vi "Live_ConvertSetting_Examples.vi"() -> ()   [LabVIEW 2019]
doc: "This example demonstrates the image acquisition with one camera in ring buffer mode together with a live display of the latest images during record. After record is stopped, the images can be addressed by index.\nAdditionally the image convert settings can be adjusted at any time\nNote that this example will not be fail save, i.e. doesnt react on errors, just handles them forward to the end\n\nUsage:\nSelect your required image count and the camera setup before you start the program.\nOnce started, the camera class will be initialized and images will be recorded and displayed automatically\nYou can stop the images by pressing stop record.\nAfter stopped, the image at the selected index will be read out\nTo finish the program click on quit application, this will force an exit of the camera class\nYou can change your required ROI after and also during the record."
uses:
  camera/Camera.lvclass
  pco.sdk/TimingControl/TimingControl.lvlib
  <vilib>/picture/picture.llb/Draw True-Color Pixmap.vi
  <vilib>/picture/picture.llb/Draw 8-Bit Pixmap.vi
panel:
  out "colormap(U8)":u32[](array[numeric])
  out "Image(U16)":u16[][](graph)
  in  "Zoom [%]":i32(slide)=26 min=10 max=200 step=5 scale=10.0..200.0
  out "Image":picture
  in  "settingsChanged":bool
  in  "Trigger":bool
  in  "LUT File":path
  in  "data_format":T1(ring)=enum."RGBA8"
  in  "Auto Range":bool
  out "rawImage":u16[][](array[numeric])
  in  "iContrast [%]":i32 min=-100 max=99 step=1
  in  "Gamma":dbl=1.0 min=0.01 max=10.0 step=0.01 format="%.2f"
  in  "whiteBalance":bool
  in  "iScale_max":u16=60000 step=1
  in  "iScale_min":u16=200 step=1
  in  "Image Index":u32 max=9
  out "Recorded Images":u32
  in  "TriggerMode":T2(ring)
  in  "Quit":bool
  out "Error":errorcluster {"code" format="%x"}
  in  "Stop Record":bool
  out "Recording On":bool
  in  "cropY1":u64=2 min=1 max=2048 step=1
  in  "cropX1":u64=2 min=1 max=2048 step=1
  in  "cropY0":u64=1 min=1 max=2047 step=1
  in  "cropX0":u64=1 min=1 max=2047 step=1
  out "Image Height":u64
  out "Image Width":u64
  in  "dwImgCount":u32=10 caption="Required Number of Images" max=2397
  in  "Exposure Time [s]":dbl=0.010000000000000002 step=0.001
  # "This example demonstrates the image acquisition with one camera in ring buffer mode together with a live display of the latest images during record. After record is stopped, the images can be addressed by index.\nAdditionally the image convert settings can be adjusted at any time\nNote that this example will not be fail save, i.e. doesnt react on errors, just handles them forward to the end\n\nUsage:\nSelect your required image count and the camera setup before you start the program.\nOnce started, the camera class will be initialized and images will be recorded and displayed automatically\nYou can stop the images by pressing stop record.\nAfter stopped, the image at the selected index will be read out\nTo finish the program click on quit application, this will force an exit of the camera class\nYou can change your required ROI after and also during the record."
  # "pco.labview"
  # "Camera Setup"
  # "Recording Control"
  # "Parameters for image readout"
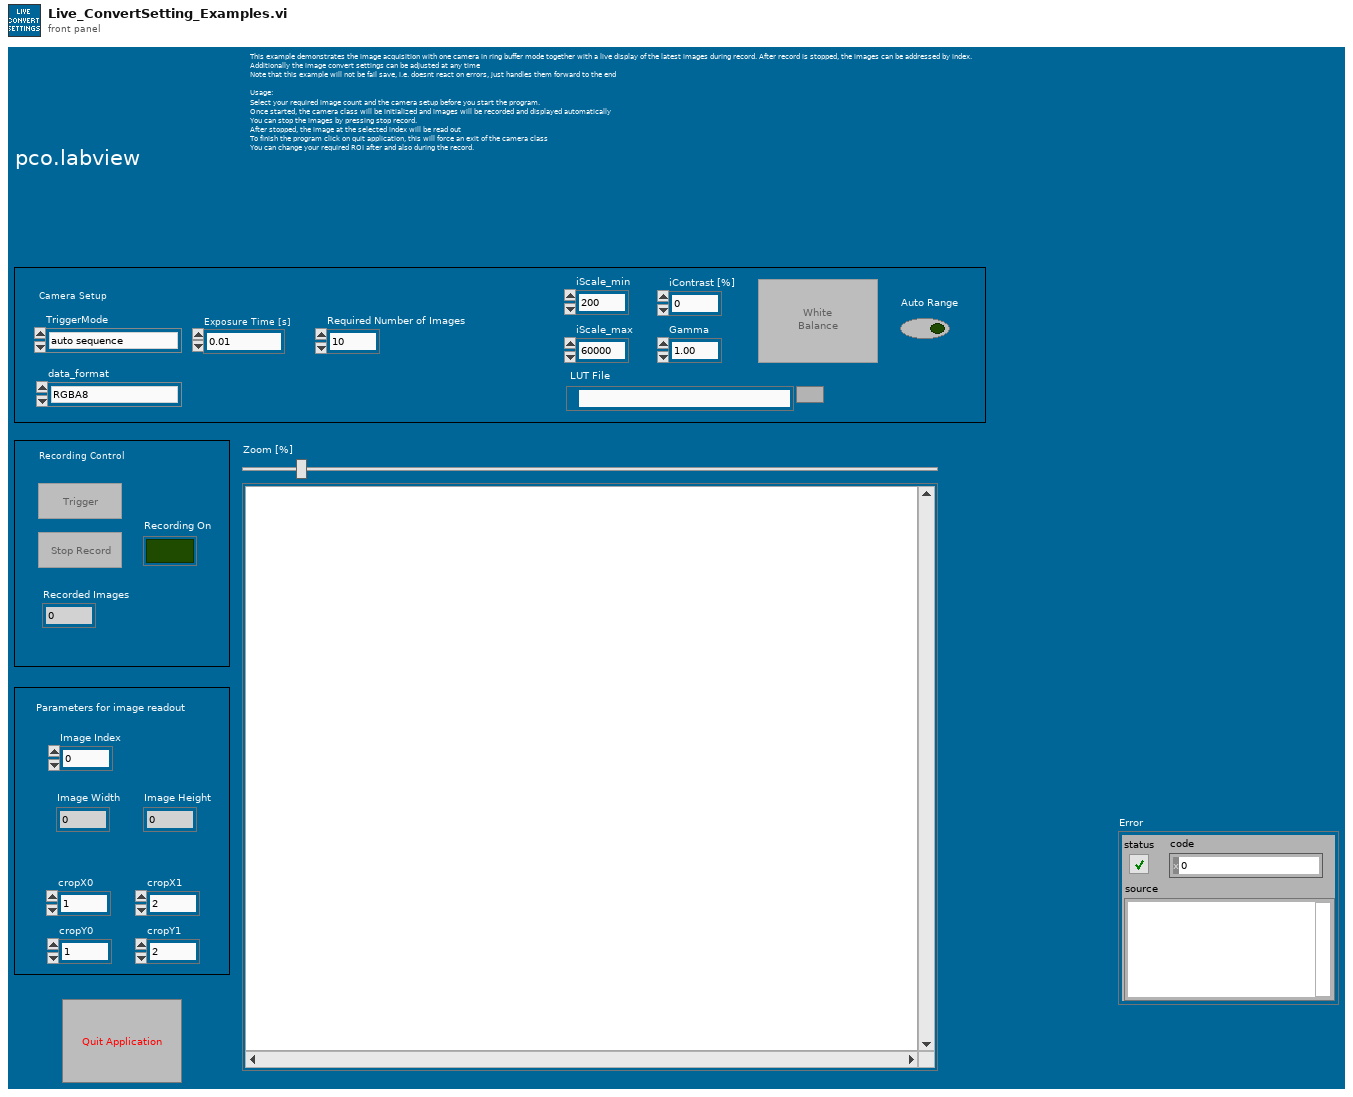
[diagram p1: front panel]
types:
  T1 = enum16{"Undefined", "Mono8", "Mono16", "BGRA8", "RGBA8", "BGRA16", "RGBA16", "CompressedMono8"}
  T2 = enum16{"auto sequence", "software trigger", "external exposure start", "external exposure control"}
  T3 = enum16{"sequence", "sequence non blocking", "ring buffer", "fifo", "tif", "multitif", "pcoraw", "b16", "dicom", "multidicom", "camram_ring", "camram_segment"}
  T4 = enum8{"Enabled", "Disabled", "Disabled and Grayed Out"}
  T5 = cluster{"serial":u32, "type":u16, "sub_type":u16, "interface_type":u16, "bit_resolution":u16, "min_exposure_time_s":dbl, "max_exposure_time_s":dbl, "min_exposure_step_s":dbl, "min_delay_time_s":dbl, "max_delay_time_s":dbl, "min_delay_step_s":dbl, "min_width":u64, "min_height":u64, "max_width":u64, "max_height":u64, "roi_step_horz":u64, "roi_step_vert":u64, "roi_symmetric_horz":bool, "roi_symmetric_vert":bool, "has_timestamp_mode":bool, "has_timestamp_mode_ascii_only":bool, "pixelrate_vec":u32[], "conversion_factor_vec":sgl[], "has_trigger_mode_extexpctrl":bool, "has_acquire_mode":bool, "has_ext_acquire_mode":bool, "has_metadata_mode":bool, "has_ram":bool, "binning_horz_vec":u16[], "binning_vert_vec":u16[], "has_average_binning":bool, "pixel_format_vec":u32[]}
  T6 = cluster{"wSignalNum":u16, "wEnabled":u16, "wType":u16, "wPolarity":u16, "wFilterSetting":u16, "wSelected":u16, "dwParameter":u32[], "dwSignalFunctionality":u32[]}
  T7 = typedef "Camera.lvclass/binning.ctl" = cluster{"vert":u16, "horz":u16, "mode":u16}
  T8 = cluster{"exposure_time_s":dbl, "delay_time_s":dbl, "roi":cluster{"x0":u64, "y0":u64, "x1":u64, "y1":u64}, "timestamp_mode":u16, "pixelrate":u32, "conversion_factor":sgl, "trigger_mode":u16, "acquire_mode":u16, "acquire_sequence_number":u32, "metadata_mode":u16, "noisefilter_mode":u16, "pixel_format":u32, "binning":T7, "auto_exposure":cluster{"region":u16, "min_exposure_s":dbl, "max_exposure_s":dbl}}
  T9 = cluster{"sharpen":bool, "adaptive_sharpen":bool, "flip_vertical":bool, "auto_minmax":bool, "add_conv_flags":u32, "min_limit":u16, "max_limit":u16, "gamma":dbl, "contrast":i32, "pco_debayer_algorithm":bool, "color_temperature":i32, "color_saturation":i32, "color_vibrance":i32, "color_tint":i32, "lut_file":path}
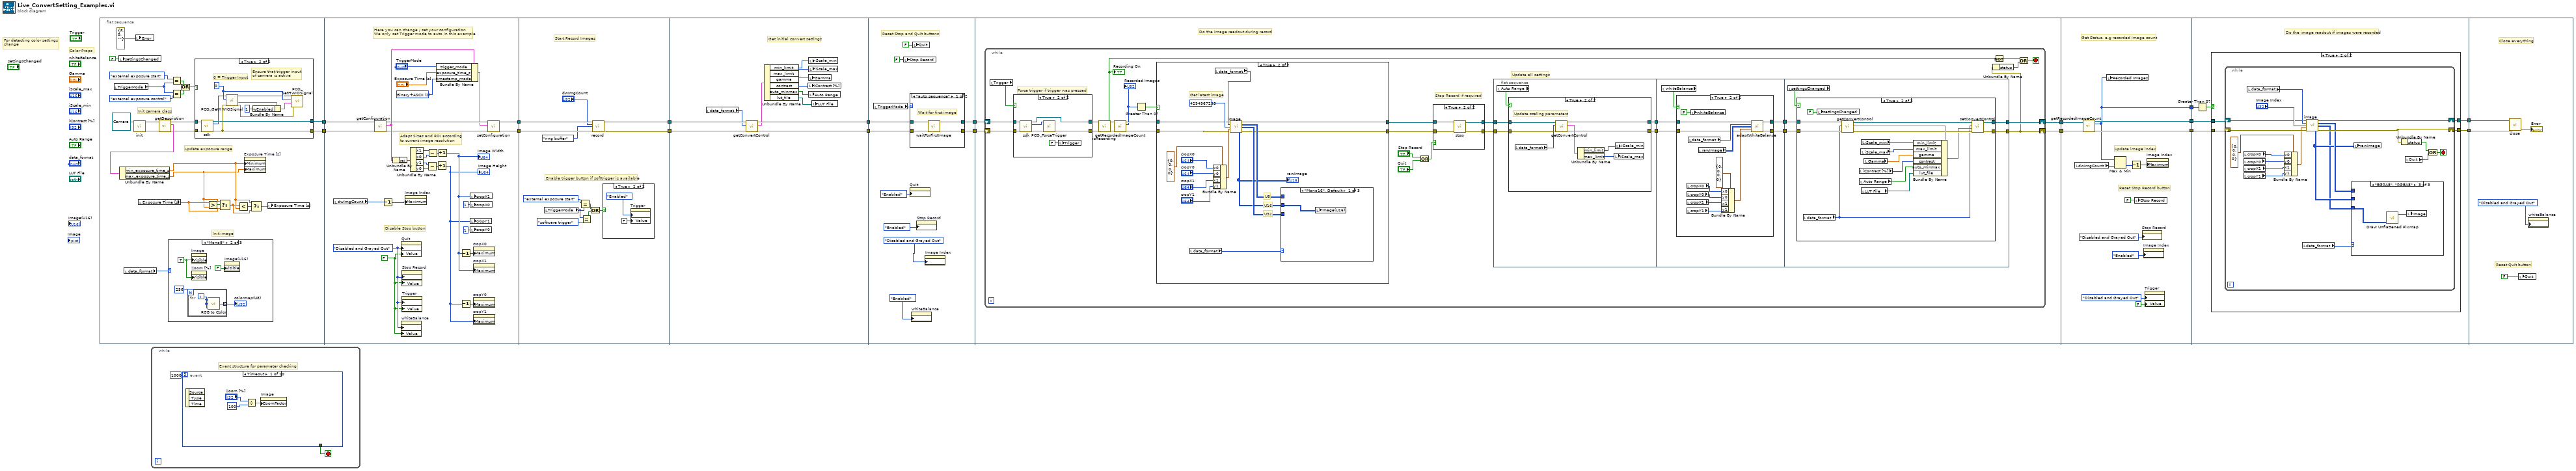
[diagram p0: block diagram]
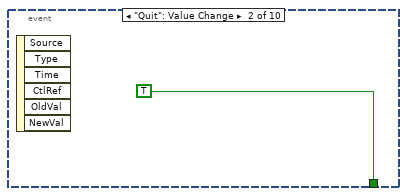
[diagram p2: hidden frame]
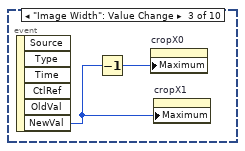
[diagram p3: hidden frame]
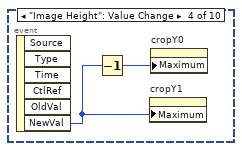
[diagram p4: hidden frame]
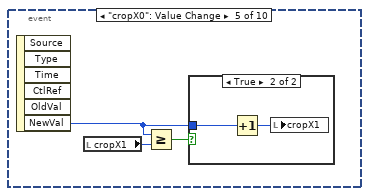
[diagram p5: hidden frame]
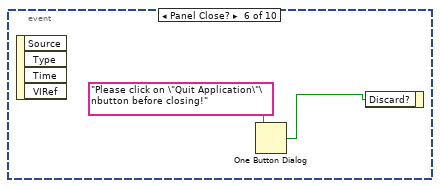
[diagram p7: hidden frame]
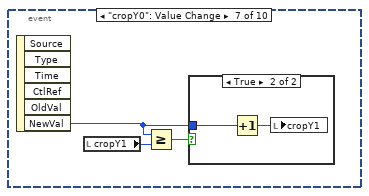
[diagram p8: hidden frame]
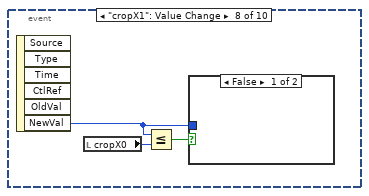
[diagram p10: hidden frame]
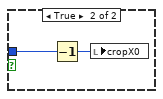
[diagram p11: hidden frame]
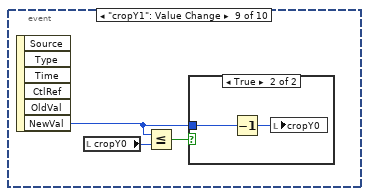
[diagram p12: hidden frame]
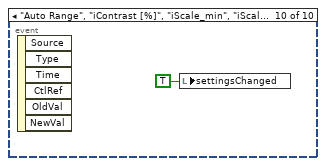
[diagram p14: hidden frame]
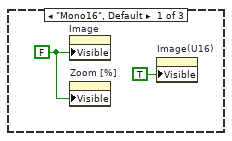
[diagram p16: hidden frame]
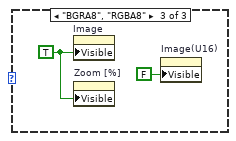
[diagram p17: hidden frame]
diagram:
  # "For detecting color settings\nchange"
  # "Color Props"
  n1 = flat-sequence {
    tunnel: [w24] -> w7
    tunnel: [w25] -> w1
    tunnel: [w69] -> w17
    tunnel: [w73] -> w16
    tunnel: w7 -> [w68]
    tunnel: w1 -> [w67]
    tunnel: w17 -> [w103]
    tunnel: w16 -> [w104]
    tunnel: [w100] -> w11
    tunnel: [w101] -> w8
    tunnel: w11 -> [w117]
    tunnel: [w112] -> w10
    tunnel: [w118] -> w9
    tunnel: w8 -> [w108]
    tunnel: w10 -> [w125]
    tunnel: w9 -> [w126]
    tunnel: [w124] -> w15
    tunnel: [w121] -> w3
    tunnel: w15 -> [w139]
    tunnel: [w138] -> w14
    tunnel: [w137] -> w6
    tunnel: w3 -> [w136]
    tunnel: w14 -> [w274]
    tunnel: [w272] -> w13
    tunnel: w6 -> [w267]
    tunnel: [w266] -> w5
    tunnel: [w265] -> w2
    tunnel: w13 -> [w283]
    tunnel: [w282] -> w12
    tunnel: w5 -> [w281]
    tunnel: [w280] -> w4
    tunnel: w2 -> [w278]
    tunnel: w12 -> [w318]
    tunnel: w4 -> [w315]
    frame #0 {
      # "Init image"
      # "Init camera class"
      # "Update exposure range"
      n2 = local read "TriggerMode"() -> (w18:T2)
      n3 = local write "settingsChanged"(FALSE ("settingsChanged")) -> ()
      n4 = local read "data_format"() -> (w29:T1)
      n5 = call-dynamic "init.vi"("Camera in"=refnum<class "Camera.lvclass"> refnum) -> ("Camera out"=w33:refnum<class "Camera.lvclass">, "error out"=w34:errorcluster)  [unwired: 8 in]
      n6 = local write "Error"(errorcluster {"status"=FALSE, "code"=0, "source"=""} ("error IO")) -> ()
      n7 = local read "Exposure Time [s]"() -> (w40:dbl)
      n8 = call-dynamic "getDescription.vi"("error in (no error)"=w34, "Camera in"=w33) -> ("error out"=w26:errorcluster, "description"=w32:T5, "Camera out"=w27:refnum<class "Camera.lvclass">)  [unwired: 7 in]
      n9 = Unbundle By Name(w32) -> ("min_exposure_time_s"=w31:dbl, "max_exposure_time_s"=w30:dbl)
      n10 = case shown="\"Mono8\"" w29 {
        frame "Mono16", Default {
          w55 = FALSE ("Visible")
          n11 = property on="Image" class="Pict"("Visible"=w55) -> ()  [unwired: 2 in, 2 out]
          n12 = property on="Zoom [%]" class="Slide (strict)"("Visible"=w55) -> ()  [unwired: 2 in, 2 out]
          n13 = property on="Image(U16)" class="IntGraph (strict)"("Visible"=TRUE) -> ()  [unwired: 2 in, 2 out]
        }
        frame "Mono8" {
          w57 = TRUE ("Visible")
          n14 = for {
            N: 256 -> [_]
            tunnel: [w61] -> w60 mode=indexing
            i -> [w62]
            n15 = call <vilib>:"RGB to Color.vi"("B"=w62, "G"=w62, "R"=w62) -> ("Color"=w61:u32)
          }
          "colormap(U8)" <- w60
          n16 = property on="Image" class="Pict"("Visible"=w57) -> ()  [unwired: 2 in, 2 out]
          n17 = property on="Zoom [%]" class="Slide (strict)"("Visible"=w57) -> ()  [unwired: 2 in, 2 out]
          n18 = property on="Image(U16)" class="IntGraph (strict)"("Visible"=FALSE) -> ()  [unwired: 2 in, 2 out]
        }
        frame "BGRA8", "RGBA8" {
          w63 = TRUE ("Visible")
          n19 = property on="Image" class="Pict"("Visible"=w63) -> ()  [unwired: 2 in, 2 out]
          n20 = property on="Zoom [%]" class="Slide (strict)"("Visible"=w63) -> ()  [unwired: 2 in, 2 out]
          n21 = property on="Image(U16)" class="IntGraph (strict)"("Visible"=FALSE) -> ()  [unwired: 2 in, 2 out]
        }
      }
      n22 = Equal?(x=T2."external exposure start" ("TriggerMode"), y=w18) -> (x = y?=w22:bool)
      n23 = Equal?(x=w18, y=T2."external exposure control" ("TriggerMode")) -> (x = y?=w21:bool)
      n24 = Or(x=w22, y=w21) -> (x .or. y?=w20:bool)
      n25 = case shown="True" w20 {
        tunnel: w27 -> [w43 w47]
        tunnel: w26 -> [w42 w46]
        tunnel: [w42 w44] -> w25
        tunnel: [w43 w45] -> w24
        frame False {
        }
        frame True {
          w52 = u16 0 ("wSignalNum")
          # "0 = Trigger Input"
          # "Ensure that trigger input\nof camera is active"
          n26 = call-dynamic "sdk.vi"("Camera in"=w47, "error in (no error)"=w46) -> ("Camera out"=w45:refnum<class "Camera.lvclass">, "sdk"=w48:u64, "error out"=w44:errorcluster)  [unwired: 11 in]
          n27 = call "PCO_GetHWIOSignal.vi"("error in (no error)"=w44, "wSignalNum"=w52, "ph"=w48) -> ("error out"=w50:errorcluster, "strSignal"=w54:T6, "ph out"=w49:u64)  [unwired: 5 in, 1 out]
          n28 = Bundle By Name(cluster=w54, "wEnabled"=u16 1) -> (w51:T6)
          n29 = call "PCO_SetHWIOSignal.vi"("error in (no error)"=w50, "strSignal"=w51, "wSignalNum"=w52, "ph"=w49) -> ()  [unwired: 5 in, 3 out]
        }
      }
      n30 = Greater?(x=w40, y=w30) -> (0:w41:bool)
      n31 = Select(t=w30, s=w41, f=w40) -> (s? t:f=w38:dbl)
      n32 = Less?(x=w38, y=w31) -> (x < y?=w39:bool)
      n33 = property on="Exposure Time [s]" class="DigNum (strict)"("Minimum"=w31, "Maximum"=w30) -> ()  [unwired: 2 in, 2 out]
      n34 = Select(t=w31, s=w39, f=w38) -> (s? t:f=w37:dbl)
      n35 = local write "Exposure Time [s]"(w37) -> ()
    }
    frame #1 {
      w79 = u16 2 items=["OFF", "Binary", "Binary+ASCII", "ASCII"] ("wTimeStampMode")
      w65 = FALSE ("Stop")
      w66 = T4."Disabled and Grayed Out" ("Disabled")
      # "Disable Stop button"
      # "Adapt Sizes and ROI according\nto current image resolution"
      # "Here you can change / set your configuration\nWe only set Trigger mode to auto in this example"
      n36 = local read "dwImgCount"() -> (w80:u32)
      n37 = call-dynamic "getConfiguration.vi"("error in (no error)"=w67, "Camera in"=w68) -> ("error out"=w74:errorcluster, "configuration"=w85:T8, "Camera out"=w76:refnum<class "Camera.lvclass">)  [unwired: 7 in]
      n38 = Decrement(x=w80) -> (x-1=w70:u32)
      n39 = Unbundle By Name(w85) -> ("roi"=w86:cluster{"x0":u64, "y0":u64, "x1":u64, "y1":u64})
      n40 = property on="Quit" class="Bool (strict)"("DisabledEnum"=w66, "Value"=w65) -> ()  [unwired: 2 in, 2 out]
      n41 = property on="whiteBalance" class="Bool (strict)"("DisabledEnum"=w66, "Value"=w65) -> ()  [unwired: 2 in, 2 out]
      n42 = property on="Stop Record" class="Bool (strict)"("DisabledEnum"=w66, "Value"=w65) -> ()  [unwired: 2 in, 2 out]
      n43 = property on="Trigger" class="Bool (strict)"("DisabledEnum"=w66, "Value"=w65) -> ()  [unwired: 2 in, 2 out]
      n44 = property on="Image Index" class="DigNum (strict)"("Maximum"=w70) -> ()  [unwired: 2 in, 2 out]
      n45 = Unbundle By Name(w86) -> ("x1"=w88:u64, "x0"=w87:u64, "y1"=w90:u64, "y0"=w89:u64)
      n46 = Subtract(x=w90, y=w89) -> (x-y=w92:u64)
      n47 = Subtract(x=w88, y=w87) -> (x-y=w91:u64)
      n48 = Bundle By Name(cluster=w85, "trigger_mode"="TriggerMode", "exposure_time_s"="Exposure Time [s]", "timestamp_mode"=w79) -> (w75:T8)
      n49 = Increment(x=w92) -> (x+1=w71:u64)
      "Image Height" <- w71
      n50 = Increment(x=w91) -> (x+1=w72:u64)
      "Image Width" <- w72
      n51 = Decrement(x=w72) -> (x-1=w83:u64)
      n52 = Decrement(x=w71) -> (x-1=w84:u64)
      n53 = local write "cropX1"(w72) -> ()
      n54 = local write "cropX0"(u64 1 ("roiY0")) -> ()
      n55 = local write "cropY1"(w71) -> ()
      n56 = local write "cropY0"(u64 1 ("roiY0")) -> ()
      n57 = property on="cropX0" class="DigNum (strict)"("Maximum"=w83) -> ()  [unwired: 2 in, 2 out]
      n58 = property on="cropX1" class="DigNum (strict)"("Maximum"=w72) -> ()  [unwired: 2 in, 2 out]
      n59 = property on="cropY0" class="DigNum (strict)"("Maximum"=w84) -> ()  [unwired: 2 in, 2 out]
      n60 = property on="cropY1" class="DigNum (strict)"("Maximum"=w71) -> ()  [unwired: 2 in, 2 out]
      n61 = call-dynamic "setConfiguration.vi"("error in (no error)"=w74, "configuration"=w75, "Camera in"=w76) -> ("error out"=w73:errorcluster, "Camera out"=w69:refnum<class "Camera.lvclass">)  [unwired: 7 in]
    }
    frame #2 {
      # "Enable trigger button if softtrigger is available"
      # "Start Record Images"
      n62 = local read "TriggerMode"() -> (w98:T2)
      n63 = Equal?(x=T2."external exposure start" ("TriggerMode"), y=w98) -> (x = y?=w95:bool)
      n64 = Equal?(x=w98, y=T2."software trigger" ("TriggerMode")) -> (x = y?=w94:bool)
      n65 = Or(x=w95, y=w94) -> (x .or. y?=w96:bool)
      n66 = call-dynamic "record.vi"("Camera in"=w103, "num_images"="dwImgCount", "record_mode"=T3."ring buffer", "error in (no error)"=w104) -> ("Camera out"=w101:refnum<class "Camera.lvclass">, "error out"=w100:errorcluster)  [unwired: 10 in]
      n67 = case shown="True" w96 {
        frame False {
        }
        frame True {
          n68 = property on="Trigger" class="Bool (strict)"("DisabledEnum"=T4."Enabled" ("Disabled"), "Value"=FALSE ("Trigger")) -> ()  [unwired: 2 in, 2 out]
        }
      }
    }
    frame #3 {
      # "Get initial convert settings"
      n69 = local read "data_format"() -> (w107:T1)
      n70 = call-dynamic "getConvertControl.vi"("error in (no error)"=w117, "data_format"=w107, "Camera in"=w108) -> ("error out"=w112:errorcluster, "convert_control"=w116:T9, "Camera out"=w118:refnum<class "Camera.lvclass">)  [unwired: 6 in]
      n71 = Unbundle By Name(w116) -> ("min_limit"=w114:u16, "max_limit"=w113:u16, "gamma"=w115:dbl, "contrast"=w111:i32, "auto_minmax"=w110:bool, "lut_file"=w109:path)
      n72 = local write "iContrast [%]"(w111) -> ()
      n73 = local write "Gamma"(w115) -> ()
      n74 = local write "iScale_min"(w114) -> ()
      n75 = local write "iScale_max"(w113) -> ()
      n76 = local write "Auto Range"(w110) -> ()
      n77 = local write "LUT File"(w109) -> ()
    }
    frame #4 {
      # "Reset Stop and Quit buttons"
      n78 = local read "TriggerMode"() -> (w119:T2)
      n79 = local write "Stop Record"(FALSE ("Stop Record")) -> ()
      n80 = case shown="\"auto sequence\"" w119 {
        tunnel: w126 -> [w133 w135]
        tunnel: w125 -> [w132 w134]
        tunnel: [w131 w134] -> w124
        tunnel: [w130 w135] -> w121
        frame "auto sequence" {
          # "Wait for first image"
          n81 = call-dynamic "waitForFirstImage.vi"("error in (no error)"=w132, "Camera in"=w133) -> ("error out"=w131:errorcluster, "Camera out"=w130:refnum<class "Camera.lvclass">)  [unwired: 8 in]
        }
        frame Default {
          # "Don't wait \nif we trigger"
        }
      }
      n82 = property on="Quit" class="Bool (strict)"("DisabledEnum"=T4."Enabled" ("Disabled")) -> ()  [unwired: 2 in, 2 out]
      n83 = property on="whiteBalance" class="Bool (strict)"("DisabledEnum"=T4."Enabled" ("Disabled")) -> ()  [unwired: 2 in, 2 out]
      n84 = local write "Quit"(FALSE ("Stop")) -> ()
      n85 = property on="Stop Record" class="Bool (strict)"("DisabledEnum"=T4."Enabled" ("Disabled")) -> ()  [unwired: 2 in, 2 out]
      n86 = property on="Image Index" class="DigNum (strict)"("DisabledEnum"=T4."Disabled and Grayed Out" ("Disabled")) -> ()  [unwired: 2 in, 2 out]
    }
    frame #5 {
      # "Do the image readout during record"
      n87 = while {
        shift-right: [w149] -> w138
        shift-left: w139 -> [w152]
        shift-right: [w155] -> w137
        shift-left: w136 -> [w153]
        stop <- w167 stop-if-true
        # "Stop Record if required"
        # "Force trigger if trigger was pressed"
        # "Update all settings"
        n88 = local read "Trigger"() -> (w154:bool)
        n89 = case shown="True" w154 {
          tunnel: w153 -> [w199 w204]
          tunnel: w152 -> [w198 w203]
          tunnel: [w199 w202] -> w151
          tunnel: [w198 w201] -> w150
          frame False {
          }
          frame True {
            n90 = call-dynamic "sdk.vi"("Camera in"=w204, "error in (no error)"=w203) -> ("Camera out"=w202:refnum<class "Camera.lvclass">, "sdk"=w205:u64, "error out"=w206:errorcluster)  [unwired: 11 in]
            n91 = call "PCO_ForceTrigger.vi"("error in (no error)"=w206, "ph"=w205) -> ("error out"=w201:errorcluster)  [unwired: 6 in, 3 out]
            n92 = local write "Trigger"(FALSE ("Trigger")) -> ()
          }
        }
        n93 = call-dynamic "isRecording.vi"("Camera in"=w151, "error in (no error)"=w150) -> ("Camera out"=w163:refnum<class "Camera.lvclass">, "recording"=w165:bool, "error out"=w162:errorcluster)  [unwired: 11 in]
        "Recording On" <- w165
        n94 = call-dynamic "getRecordedImageCount.vi"("Camera in"=w163, "error in (no error)"=w162) -> ("Camera out"=w160:refnum<class "Camera.lvclass">, "recorded_image_count"=w148:u32, "error out"=w161:errorcluster)  [unwired: 11 in]
        "Recorded Images" <- w148
        n95 = Greater Than 0?(x=w148) -> (x > 0?=w147:bool)
        n96 = case shown="True" w147 {
          tunnel: w161 -> [w174 w184]
          tunnel: w160 -> [w175 w178]
          tunnel: [w174 w176] -> w143
          tunnel: [w175 w177] -> w142
          frame False {
          }
          frame True {
            # "U32"
            # "U8"
            # "U16"
            # "Get latest image"
            n97 = local read "data_format"() -> (w179:T1)
            n98 = Bundle By Name(cluster=cluster{"x0":u64, "y0":u64, "x1":u64, "y1":u64} {"x0"=0, "y0"=0, "x1"=0, "y1"=0} ("roi"), "x0"="cropX0", "y0"="cropY0", "x1"="cropX1", "y1"="cropY1") -> (w187:cluster{"x0":u64, "y0":u64, "x1":u64, "y1":u64})
            n99 = local read "data_format"() -> (w183:T1)
            n100 = call-dynamic "image.vi"("Camera in"=w178, "data_format"=w183, "image_index"=u32 4294967295 ("dwImgIdx"), "crop"=w187, "error in (no error)"=w184) -> ("Camera out"=w177:refnum<class "Camera.lvclass">, "image (U8)"=w181:u8[][], "image (U32)"=w182:u32[][], "raw_image (U16)"=w180:u16[][], "error out"=w176:errorcluster)  [unwired: 2 in, 4 out]
            "rawImage" <- w180
            n101 = case shown="\"Mono16\", Default" w179 {
              tunnel: w182 -> [_ _ w197]
              tunnel: w181 -> [_ w194 _]
              tunnel: w180 -> [w192 _ _]
              frame "Mono16", Default {
                n102 = local write "Image(U16)"(w192) -> ()
              }
              frame "Mono8" {
                n103 = local read "colormap(U8)"() -> (w193:u32[])
                n104 = call-poly <vilib>:"Draw Unflattened Pixmap.vi"("data"=w194, "color table"=w193) -> ("new picture"=w195:picture)  [unwired: 7 in]
                n105 = local write "Image"(w195) -> ()
              }
              frame "BGRA8", "RGBA8" {
                n106 = call-poly <vilib>:"Draw Unflattened Pixmap.vi"("data (RGB format)"=w197) -> ("new picture"=w196:picture)  [unwired: 8 in]
                n107 = local write "Image"(w196) -> ()
              }
            }
          }
        }
        n108 = Or(x="Stop Record", y="Quit") -> (x .or. y?=w146:bool)
        n109 = case shown="True" w146 {
          tunnel: w143 -> [w169 w170]
          tunnel: [w168 w172] -> w141
          tunnel: [w169 w173] -> w140
          tunnel: w142 -> [w168 w171]
          frame False {
          }
          frame True {
            n110 = call-dynamic "stop.vi"("error in (no error)"=w170, "Camera in"=w171) -> ("error out"=w173:errorcluster, "Camera out"=w172:refnum<class "Camera.lvclass">)  [unwired: 8 in]
          }
        }
        n111 = flat-sequence {
          tunnel: w140 -> [w209]
          tunnel: w141 -> [w210]
          tunnel: [w208] -> w159
          tunnel: [w207] -> w158
          tunnel: w159 -> [w225]
          tunnel: w158 -> [w224]
          tunnel: [w223] -> w157
          tunnel: [w222] -> w156
          tunnel: w157 -> [w244]
          tunnel: w156 -> [w245]
          tunnel: [w243] -> w149
          tunnel: [w242] -> w155
          frame #0 {
            n112 = local read "Auto Range"() -> (w211:bool)
            n113 = case shown="True" w211 {
              tunnel: w210 -> [w213 w217]
              tunnel: w209 -> [w212 w216]
              tunnel: [w212 w215] -> w208
              tunnel: [w213 w214] -> w207
              frame False {
              }
              frame True {
                # "Update scaling parameters"
                n114 = local read "data_format"() -> (w221:T1)
                n115 = call-dynamic "getConvertControl.vi"("error in (no error)"=w216, "data_format"=w221, "Camera in"=w217) -> ("error out"=w215:errorcluster, "convert_control"=w218:T9, "Camera out"=w214:refnum<class "Camera.lvclass">)  [unwired: 6 in]
                n116 = Unbundle By Name(w218) -> ("min_limit"=w219:u16, "max_limit"=w220:u16)
                n117 = local write "iScale_max"(w220) -> ()
                n118 = local write "iScale_min"(w219) -> ()
              }
            }
          }
          frame #1 {
            n119 = local read "whiteBalance"() -> (w226:bool)
            n120 = case shown="True" w226 {
              tunnel: w225 -> [w227 w233]
              tunnel: w224 -> [w228 w232]
              tunnel: [w227 w231] -> w223
              tunnel: [w228 w230] -> w222
              frame False {
              }
              frame True {
                n121 = local read "cropX0"() -> (w238:u64)
                n122 = local read "cropY0"() -> (w237:u64)
                n123 = local read "cropX1"() -> (w236:u64)
                n124 = local read "cropY1"() -> (w229:u64)
                n125 = local read "data_format"() -> (w240:T1)
                n126 = local write "whiteBalance"(FALSE ("whiteBalance")) -> ()
                n127 = local read "rawImage"() -> (w239:u16[][])
                n128 = Bundle By Name(cluster=cluster{"x0":u64, "y0":u64, "x1":u64, "y1":u64} {"x0"=0, "y0"=0, "x1"=0, "y1"=0} ("roi"), "x0"=w238, "y0"=w237, "x1"=w236, "y1"=w229) -> (w235:cluster{"x0":u64, "y0":u64, "x1":u64, "y1":u64})
                n129 = call-dynamic "adaptWhiteBalance.vi"("Camera in"=w232, "data_format"=w240, "raw_image (U16)"=w239, "roi"=w235, "error in (no error)"=w233) -> ("Camera out"=w230:refnum<class "Camera.lvclass">, "error out"=w231:errorcluster)  [unwired: 9 in]
              }
            }
          }
          frame #2 {
            n130 = local read "settingsChanged"() -> (w246:bool)
            n131 = case shown="True" w246 {
              tunnel: w245 -> [w248 w254]
              tunnel: w244 -> [w247 w253]
              tunnel: [w247 w250] -> w243
              tunnel: [w248 w249] -> w242
              frame False {
              }
              frame True {
                n132 = local read "data_format"() -> (w252:T1)
                n133 = local write "settingsChanged"(FALSE ("whiteBalance")) -> ()
                n134 = call-dynamic "getConvertControl.vi"("error in (no error)"=w253, "data_format"=w252, "Camera in"=w254) -> ("error out"=w256:errorcluster, "convert_control"=w263:T9, "Camera out"=w257:refnum<class "Camera.lvclass">)  [unwired: 6 in]
                n135 = local read "iContrast [%]"() -> (w259:i32)
                n136 = local read "Auto Range"() -> (w258:bool)
                n137 = local read "iScale_max"() -> (w261:u16)
                n138 = local read "iScale_min"() -> (w262:u16)
                n139 = local read "LUT File"() -> (w251:path)
                n140 = local read "Gamma"() -> (w260:dbl)
                n141 = Bundle By Name(cluster=w263, "min_limit"=w262, "max_limit"=w261, "gamma"=w260, "contrast"=w259, "auto_minmax"=w258, "lut_file"=w251) -> (w255:T9)
                n142 = call-dynamic "setConvertControl.vi"("error in (no error)"=w256, "convert_control"=w255, "data_format"=w252, "Camera in"=w257) -> ("error out"=w250:errorcluster, "Camera out"=w249:refnum<class "Camera.lvclass">)  [unwired: 6 in]
              }
            }
          }
        }
        n143 = Unbundle By Name(w149) -> ("status"=w166:bool)
        n144 = Not(x=w165) -> (.not. x?=w164:bool)
        n145 = Or(x=w164, y=w166) -> (x .or. y?=w167:bool)
      }
    }
    frame #6 {
      # "Update image index"
      # "Reset Stop Record button"
      # "Get Status, e.g recorded image count"
      n146 = local read "dwImgCount"() -> (w273:u32)
      n147 = call-dynamic "getRecordedImageCount.vi"("Camera in"=w267, "error in (no error)"=w274) -> ("Camera out"=w266:refnum<class "Camera.lvclass">, "recorded_image_count"=w265:u32, "error out"=w272:errorcluster)  [unwired: 11 in]
      n148 = local write "Recorded Images"(w265) -> ()
      n149 = Max & Min(x=w265, y=w273) -> (min(x,y)=w275:u32)  [unwired: 1 out]
      n150 = Decrement(x=w275) -> (x-1=w270:u32)
      n151 = local write "Stop Record"(FALSE ("Stop Record")) -> ()
      n152 = property on="Stop Record" class="Bool (strict)"("DisabledEnum"=T4."Disabled and Grayed Out" ("Disabled")) -> ()  [unwired: 2 in, 2 out]
      n153 = property on="Image Index" class="DigNum (strict)"("DisabledEnum"=T4."Enabled" ("Disabled")) -> ()  [unwired: 2 in, 2 out]
      n154 = property on="Trigger" class="Bool (strict)"("DisabledEnum"=T4."Disabled and Grayed Out" ("Disabled"), "Value"=FALSE ("Trigger")) -> ()  [unwired: 2 in, 2 out]
      n155 = property on="Image Index" class="DigNum (strict)"("Maximum"=w270) -> ()  [unwired: 2 in, 2 out]
    }
    frame #7 {
      # "Do the image readout if images were recorded"
      n156 = Greater Than 0?(x=w278) -> (x > 0?=w279:bool)
      n157 = case shown="True" w279 {
        tunnel: w283 -> [w284 w289]
        tunnel: [w284 w288] -> w282
        tunnel: w281 -> [w285 w287]
        tunnel: [w285 w286] -> w280
        frame False {
        }
        frame True {
          n158 = while {
            shift-right: [w300] -> w288
            shift-left: w289 -> [w308]
            shift-right: [w294] -> w286
            shift-left: w287 -> [w295]
            stop <- w302 stop-if-true
            n159 = local read "cropX0"() -> (w298:u64)
            n160 = local read "cropY0"() -> (w299:u64)
            n161 = local read "cropX1"() -> (w306:u64)
            n162 = local read "cropY1"() -> (w305:u64)
            n163 = local read "data_format"() -> (w296:T1)
            n164 = Bundle By Name(cluster=cluster{"x0":u64, "y0":u64, "x1":u64, "y1":u64} {"x0"=0, "y0"=0, "x1"=0, "y1"=0} ("roi"), "x0"=w298, "y0"=w299, "x1"=w306, "y1"=w305) -> (w307:cluster{"x0":u64, "y0":u64, "x1":u64, "y1":u64})
            n165 = local read "data_format"() -> (w290:T1)
            n166 = call-dynamic "image.vi"("Camera in"=w295, "data_format"=w296, "image_index"="Image Index", "crop"=w307, "error in (no error)"=w308) -> ("Camera out"=w294:refnum<class "Camera.lvclass">, "image (U8)"=w293:u8[][], "image (U32)"=w291:u32[][], "raw_image (U16)"=w292:u16[][], "error out"=w300:errorcluster)  [unwired: 2 in, 4 out]
            n167 = case shown="\"BGRA8\", \"RGBA8\"" w290 {
              tunnel: w291 -> [_ _ w314]
              tunnel: w293 -> [_ w311 _]
              tunnel: w292 -> [w309 _ _]
              frame "Mono16", Default {
                n168 = local write "Image(U16)"(w309) -> ()
              }
              frame "Mono8" {
                n169 = local read "colormap(U8)"() -> (w310:u32[])
                n170 = call-poly <vilib>:"Draw Unflattened Pixmap.vi"("data"=w311, "color table"=w310) -> ("new picture"=w312:picture)  [unwired: 7 in]
                n171 = local write "Image"(w312) -> ()
              }
              frame "BGRA8", "RGBA8" {
                n172 = call-poly <vilib>:"Draw Unflattened Pixmap.vi"("data (RGB format)"=w314) -> ("new picture"=w313:picture)  [unwired: 8 in]
                n173 = local write "Image"(w313) -> ()
              }
            }
            n174 = local write "rawImage"(w292) -> ()
            n175 = Unbundle By Name(w300) -> ("status"=w303:bool)
            n176 = local read "Quit"() -> (w304:bool)
            n177 = Or(x=w303, y=w304) -> (x .or. y?=w302:bool)
          }
        }
      }
    }
    frame #8 {
      # "Close everything"
      # "Reset Quit button"
      n178 = call-dynamic "close.vi"("error in (no error)"=w318, "Camera in"=w315) -> ("error out"=→"Error":errorcluster)  [unwired: 9 in]
      n179 = local write "Quit"(FALSE ("Stop Record")) -> ()
      n180 = property on="whiteBalance" class="Bool (strict)"("DisabledEnum"=T4."Disabled and Grayed Out" ("Disabled")) -> ()  [unwired: 2 in, 2 out]
    }
  }
  n181 = while {
    stop <- w320 stop-if-true
    # "Event structure for parameter checking"
    n182 = event shown="[0] Timeout" {
      selector: _ -> [_ _ _ _ _ _ _ _ _ _]
      dyn-events: _ -> [_ _ _ _ _ _ _ _ _ _]
      timeout: 1000 -> [_ _ _ _ _ _ _ _ _ _]
      tunnel: [_ TRUE _ _ _ _ _ _ _ _] -> w320
      event Timeout {
        n183 = event-data() -> ()  [unwired: 1 in, 3 out]
        n184 = Divide(x="Zoom [%]", y=100 ("Zoom [%]")) -> (x/y=w324:dbl)
        n185 = property on="Image" class="Pict"("ZoomFactor"=w324) -> ()  [unwired: 2 in, 2 out]
      }
      event "Quit": Value Change {
        n186 = event-data() -> ()  [unwired: 1 in, 6 out]
      }
      event "Image Width": Value Change {
        n187 = event-data() -> ("NewVal"=w326:u64)  [unwired: 1 in, 5 out]
        n188 = Decrement(x=w326) -> (x-1=w327:u64)
        n189 = property on="cropX0" class="DigNum (strict)"("Maximum"=w327) -> ()  [unwired: 2 in, 2 out]
        n190 = property on="cropX1" class="DigNum (strict)"("Maximum"=w326) -> ()  [unwired: 2 in, 2 out]
      }
      event "Image Height": Value Change {
        n191 = event-data() -> ("NewVal"=w328:u64)  [unwired: 1 in, 5 out]
        n192 = Decrement(x=w328) -> (x-1=w329:u64)
        n193 = property on="cropY1" class="DigNum (strict)"("Maximum"=w328) -> ()  [unwired: 2 in, 2 out]
        n194 = property on="cropY0" class="DigNum (strict)"("Maximum"=w329) -> ()  [unwired: 2 in, 2 out]
      }
      event "cropX0": Value Change {
        n195 = event-data() -> ("NewVal"=w330:u64)  [unwired: 1 in, 5 out]
        n196 = local read "cropX1"() -> (w332:u64)
        n197 = Greater Or Equal?(x=w330, y=w332) -> (x >= y?=w331:bool)
        n198 = case shown="True" w331 {
          tunnel: w330 -> [_ w334]
          frame False {
          }
          frame True {
            n199 = Increment(x=w334) -> (x+1=w333:u64)
            n200 = local write "cropX1"(w333) -> ()
          }
        }
      }
      event Panel Close? {
        n201 = event-data() -> ()  [unwired: 1 in, 4 out]
        n202 = One Button Dialog(message="Please click on \"Quit Application\"\nbutton before closing!") -> (true=w335:bool)  [unwired: 1 in]
        n203 = event-data("Discard?"=w335) -> ()  [unwired: 1 in, 1 out]
      }
      event "cropY0": Value Change {
        n204 = event-data() -> ("NewVal"=w337:u64)  [unwired: 1 in, 5 out]
        n205 = local read "cropY1"() -> (w339:u64)
        n206 = Greater Or Equal?(x=w337, y=w339) -> (x >= y?=w338:bool)
        n207 = case shown="True" w338 {
          tunnel: w337 -> [_ w341]
          frame False {
          }
          frame True {
            n208 = Increment(x=w341) -> (x+1=w340:u64)
            n209 = local write "cropY1"(w340) -> ()
          }
        }
      }
      event "cropX1": Value Change {
        n210 = event-data() -> ("NewVal"=w342:u64)  [unwired: 1 in, 5 out]
        n211 = local read "cropX0"() -> (w344:u64)
        n212 = Less Or Equal?(x=w342, y=w344) -> (x <= y?=w343:bool)
        n213 = case shown="False" w343 {
          tunnel: w342 -> [_ w346]
          frame False {
          }
          frame True {
            n214 = Decrement(x=w346) -> (x-1=w345:u64)
            n215 = local write "cropX0"(w345) -> ()
          }
        }
      }
      event "cropY1": Value Change {
        n216 = event-data() -> ("NewVal"=w347:u64)  [unwired: 1 in, 5 out]
        n217 = local read "cropY0"() -> (w349:u64)
        n218 = Less Or Equal?(x=w347, y=w349) -> (x <= y?=w348:bool)
        n219 = case shown="True" w348 {
          tunnel: w347 -> [_ w351]
          frame False {
          }
          frame True {
            n220 = Decrement(x=w351) -> (x-1=w350:u64)
            n221 = local write "cropY0"(w350) -> ()
          }
        }
      }
      event "Auto Range", "iContrast [%]", "iScale_min", "iScale_max", "Gamma", "LUT File": Value Change {
        n222 = event-data() -> ()  [unwired: 1 in, 6 out]
        n223 = local write "settingsChanged"(TRUE ("settingsChanged")) -> ()
      }
    }
  }
